vi "配置.vi"() -> (2 "启用参数":T1, 3 "串口输出":refnum<visa-resource-name>)   [LabVIEW 2016, in "斯坦道多参数.lvlib"]
uses:
  <vilib>/Utility/miscctls.llb/LVPointTypeDef.ctl
panel:
  in  "关闭串口":bool
  in  "打开串口":bool
  in  "叶绿素a启用":bool
  in  "Temp":bool
  in  "Cond":bool
  in  "Turb":bool
  in  "DO":bool
  in  "pH":bool
  in  "关闭":bool
  in  "VISA资源名称":refnum<visa-resource-name>
  # "请设置串口参数"
  # "请选择要启用的参数"
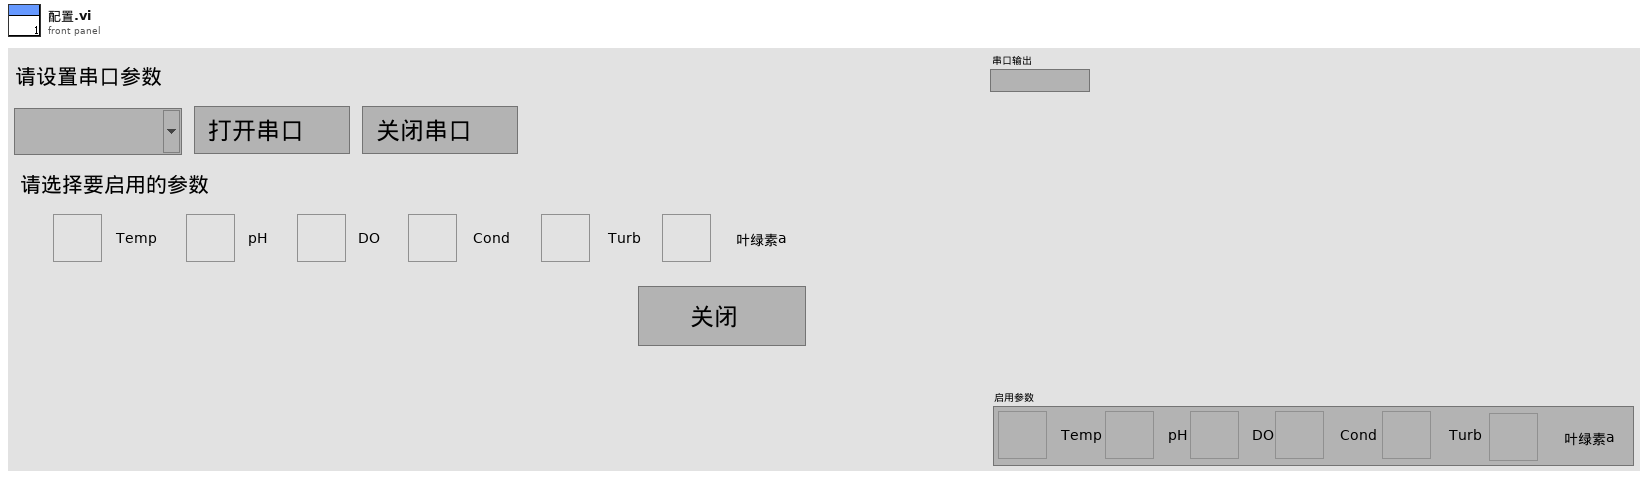
[diagram p1: front panel]
types:
  T1 = cluster{"Temp":bool, "pH":bool, "DO":bool, "Cond":bool, "Turb":bool, "叶绿素a启用":bool}
  T2 = typedef "LVPointTypeDef.ctl" = cluster{"Horizontal":i16, "Vertical":i16}
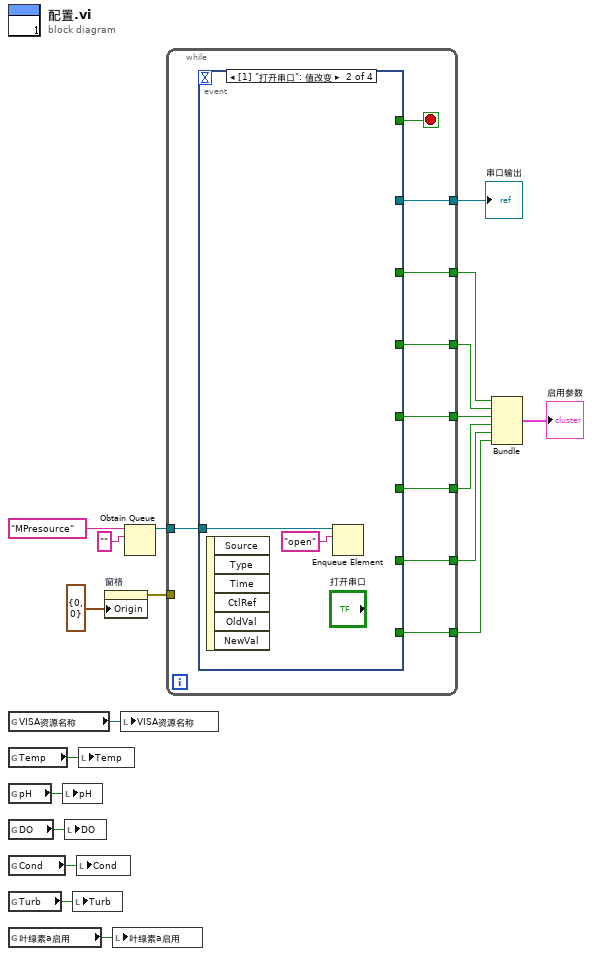
[diagram p0: block diagram]
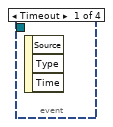
[diagram p2: hidden frame]
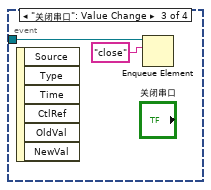
[diagram p3: hidden frame]
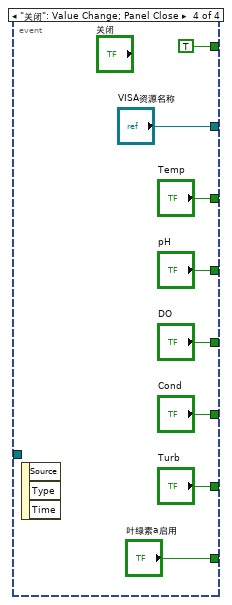
[diagram p4: hidden frame]
diagram:
  n1 = global read "断电保存变量.vi" "VISA资源名称"() -> (w13:refnum<visa-resource-name>)
  n2 = global read "断电保存变量.vi" "Temp"() -> (w8:bool)
  n3 = global read "断电保存变量.vi" "pH"() -> (w9:bool)
  n4 = global read "断电保存变量.vi" "DO"() -> (w10:bool)
  n5 = global read "断电保存变量.vi" "Cond"() -> (w11:bool)
  n6 = global read "断电保存变量.vi" "Turb"() -> (w12:bool)
  n7 = global read "断电保存变量.vi" "叶绿素a启用"() -> (w4:bool)
  n8 = local write "pH"(w9) -> ()
  n9 = local write "DO"(w10) -> ()
  n10 = local write "Turb"(w12) -> ()
  n11 = local write "Cond"(w11) -> ()
  n12 = local write "Temp"(w8) -> ()
  n13 = property on="窗格" class="Pane"("Origin"=T2 {"Horizontal"=0, "Vertical"=0} ("原点")) -> (error out=w6:errorcluster)  [unwired: 2 in, 1 out]
  n14 = local write "叶绿素a启用"(w4) -> ()
  n15 = local write "VISA资源名称"(w13) -> ()
  n16 = Obtain Queue(name (unnamed)="MPresource" ("名称（未命名）"), element data type="" ("名称（未命名）")) -> (queue out=w1:refnum<queue>)  [unwired: 3 in, 2 out]
  n17 = while {
    tunnel: [w28] -> w20
    tunnel: [w27] -> w19
    tunnel: [w26] -> w18
    tunnel: [w25] -> w17
    tunnel: [w24] -> w16
    tunnel: [w23] -> w15
    tunnel: [w22] -> w7
    tunnel: w6 -> [_]
    tunnel: w1 -> [w21]
    stop <- w29 stop-if-true
    n18 = event shown="[1] \"打开串口\": 值改变" {
      selector: _ -> [_ _ _ _]
      dyn-events: _ -> [_ _ _ _]
      timeout: _ -> [_ _ _ _]
      tunnel: [_ _ _ TRUE] -> w29
      tunnel: [_ _ _ "VISA资源名称"] -> w28
      tunnel: [_ _ _ "Temp"] -> w27
      tunnel: [_ _ _ "pH"] -> w26
      tunnel: [_ _ _ "DO"] -> w25
      tunnel: [_ _ _ "Cond"] -> w24
      tunnel: [_ _ _ "Turb"] -> w23
      tunnel: [_ _ _ "叶绿素a启用"] -> w22
      tunnel: w21 -> [_ w31 w33 _]
      event Timeout {
        n19 = event-data() -> ()  [unwired: 1 in, 3 out]
      }
      event "打开串口": Value Change {
        n20 = event-data() -> ()  [unwired: 1 in, 6 out]
        n21 = Enqueue Element(queue=w31, element="open" ("元素")) -> ()  [unwired: 2 in, 3 out]
      }
      event "关闭串口": Value Change {
        n22 = event-data() -> ()  [unwired: 1 in, 6 out]
        n23 = Enqueue Element(queue=w33, element="close" ("元素")) -> ()  [unwired: 2 in, 3 out]
      }
      event "关闭": Value Change; Panel Close {
        n24 = event-data() -> ()  [unwired: 1 in, 3 out]
      }
    }
  }
  "串口输出" <- w20
  n25 = Bundle("Temp"=w19, "pH"=w18, "DO"=w17, "Cond"=w16, "Turb"=w15, "叶绿素a启用"=w7) -> (→"启用参数":T1)  [unwired: 1 in]
